vi "SchedulerVI.vi"() -> (0 "Fehler (Ausgang)":errorcluster)   [LabVIEW 2020, in "Schedule Modul.lvlib"]
uses:
  Schedule Modul.lvlib
  Aktion Trigger Freigabe.ctl
  Aktion FGV Schedule Daten.ctl
  Aktion FGV Schedule Log.ctl
  T90/Aktion FGV Automatic Start.ctl
  Funktionstasten/Funktionstasten-Aktion.ctl
  Funktionstasten/Zustaende.ctl
  AK-Schnittstelle/AK-Schnittstelle.lvlib
  Funktionstasten/Funktionstasten.lvlib
  T90/T90.lvlib
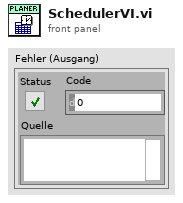
[diagram p1: front panel]
types:
  T1 = typedef "T90.lvlib/Aktion FGV Automatic Start.ctl" = enum16{"lesen", "aktivieren", "deaktivieren"}
  T2 = typedef "Schedule Modul.lvlib/Aktion FGV Schedule Log.ctl" = enum16{"lesen", "neuer Eintrag", "laden", "löschen", "Anzeige löschen"}
  T3 = typedef "Schedule Modul.lvlib/Aktion FGV Schedule Daten.ctl" = enum16{"lesen", "laden", "speichern", "schreiben"}
  T4 = typedef "Schedule Modul.lvlib/Aktion Trigger Freigabe.ctl" = enum16{"init", "lesen", "prüfen", "löschen"}
  T5 = typedef "Funktionstasten.lvlib/Zustaende.ctl" = enum16{"Standby", "Pause", "Eco", "Messen", "Kalibrieren", "Spülen Filter", "Spülen Leitung", "Umgebungsluft", "0-Gas", "Cal-Gas", "CG zu PNS", "-------------", "Init 1", "Init 2", "Init 3", "Init 4", "Messen vorbereiten", "Messen durchführen", "Exit"}
  T6 = typedef "Funktionstasten.lvlib/Funktionstasten-Aktion.ctl" = enum16{"Initialisieren", "Zustand setzen", "Taste gedrückt", "Fehler speichern", "Lesen", "Manuell", "Remote", "Bitparallel", "Samplepoint", "Zeit Prüfen", "reset Umschalten"}
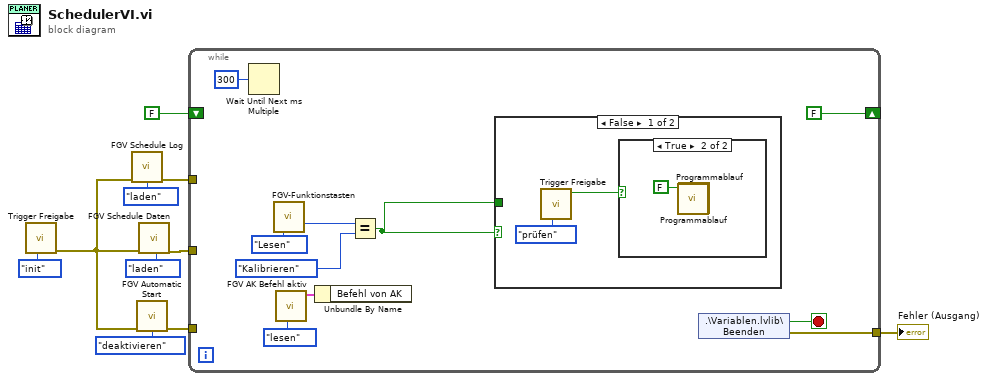
[diagram p0: block diagram]
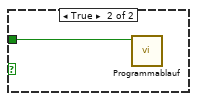
[diagram p3: hidden frame]
diagram:
  n1 = call "Trigger Freigabe.vi"("Aktion"=Aktion_Trigger_Freigabe."init") -> ("error out"=w2:errorcluster)  [unwired: 9 in, 1 out]
  n2 = call "FGV Schedule Log.vi"("error in (no error)"=w2, "Aktion"=Aktion_FGV_Schedule_Log."laden") -> ("error out"=w5:errorcluster)  [unwired: 10 in, 3 out]
  n3 = call "FGV Automatic Start.vi"("error in (no error)"=w2, "Aktion"=Aktion_FGV_Automatic_Start."deaktivieren") -> ("error out"=w1:errorcluster)  [unwired: 12 in, 1 out]
  n4 = call "FGV Schedule Daten.vi"("error in (no error)"=w2, "Aktion"=Aktion_FGV_Schedule_Daten."laden") -> ("error out"=w7:errorcluster)  [unwired: 12 in, 5 out]
  n5 = while {
    tunnel: [w19] -> w9
    tunnel: w7 -> [_]
    tunnel: w5 -> [_]
    shift-right: [FALSE] -> _
    shift-left: FALSE -> [_]
    tunnel: w1 -> [_]
    stop <- w20 stop-if-true
    n6 = Wait Until Next ms Multiple(millisecond multiple=u32 300 ("Zu wartende ms")) -> ()  [unwired: 1 out]
    n7 = call "FGV-Funktionstasten.vi"("Aktion"=Funktionstasten-Aktion."Lesen") -> ("ausgewählte Funktion"=w14:T5)  [unwired: 7 in, 7 out]
    n8 = call "FGV AK Befehl aktiv.vi"("Aktion"=enum16{"initialisieren", "lesen", "schreiben"}."lesen") -> ("Cluster (out)"=w17:cluster{"Befehl von AK":bool})  [unwired: 10 in]
    n9 = Unbundle By Name(w17) -> ()  [unwired: 1 out]
    n10 = Equal?(x=w14, y=Zustaende."Kalibrieren") -> (x = y?=w12:bool)
    n11 = case shown="False" w12 {
      tunnel: w12 -> [_ w24]
      frame False {
        n12 = call "Trigger Freigabe.vi"("Aktion"=Aktion_Trigger_Freigabe."prüfen") -> ("Freigabe"=w21:bool)  [unwired: 9 in, 1 out]
        n13 = case shown="True" w21 {
          frame False {
          }
          frame True {
            w23 = FALSE ("AK Trigger")
            n14 = call "Programmablauf.vi"("AK Trigger"=w23) -> ()  [unwired: 10 in, 1 out]
            n15 = call "Programmablauf.vi"("AK Trigger"=w23) -> ()  [unwired: 10 in, 1 out]
          }
        }
      }
      frame True {
        n16 = call "Programmablauf.vi"("AK Trigger"=w24) -> ()  [unwired: 10 in, 1 out]
      }
    }
    n17 = shared-variable ".\\Variablen.lvlib\\Beenden"() -> (w20:bool, error out=w19:errorcluster)  [unwired: 1 out]
  }
  "Fehler (Ausgang)" <- w9
